vi "Device sw.vi"(1 "Device switch":enum16{"Mouse", "Keyboard"}(ring), 2 "Auto?":bool) -> (0 "output state":T1(ring))   [LabVIEW 2019]
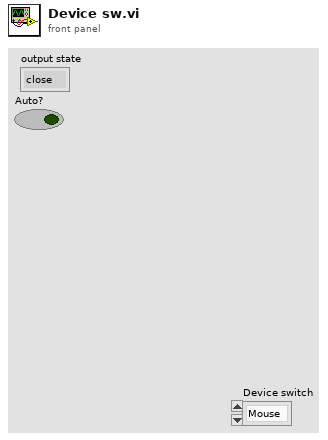
[diagram p1: front panel]
types:
  T1 = enum16{"close", "start keyboard", "start mouse", "output"}
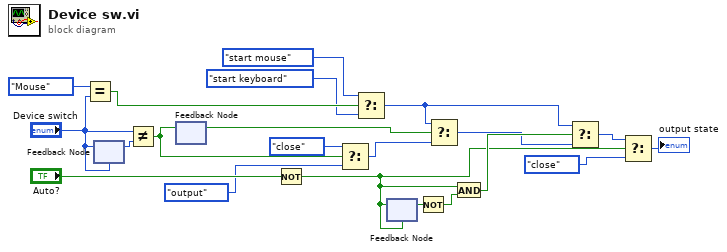
[diagram p0: block diagram]
diagram:
  n1 = Equal?(x=enum16{"Mouse", "Keyboard"}."Mouse", y="Device switch") -> (x = y?=w15:bool)
  n2 = feedback #1("Device switch") -> (w10:enum16{"Mouse", "Keyboard"})
  n3 = feedback-in #1("Device switch") -> ()
  n4 = Not Equal?(x="Device switch", y=w10) -> (x != y?=w9:bool)
  n5 = feedback #2() -> (w6:bool)  [unwired: 1 in]
  n6 = feedback-in #2(w9) -> ()
  n7 = Not(x="Auto?") -> (.not. x?=w1:bool)
  n8 = Select(t=T1."close", s=w9, f=T1."output" ("Enum")) -> (s? t:f=w4:T1)
  n9 = Select(t=T1."start mouse" ("Enum"), s=w15, f=T1."start keyboard" ("Enum")) -> (s? t:f=w3:T1)
  n10 = feedback #3(w1) -> (w19:bool)
  n11 = feedback-in #3(w1) -> ()
  n12 = Not(x=w19) -> (.not. x?=w18:bool)
  n13 = Select(t=w3, s=w6, f=w4) -> (s? t:f=w2:T1)
  n14 = And(x=w1, y=w18) -> (x .and. y?=w17:bool)
  n15 = Select(t=w3, s=w17, f=w2) -> (s? t:f=w20:T1)
  n16 = Select(t=w20, s=w1, f=T1."close" ("Enum")) -> (s? t:f=→"output state":T1)
